vi "Calculator-test_harness.vi"(11 "test case ID":string) -> (3 "result":bool)   [LabVIEW 2018]
doc: "The harness VI is executed for every test case. InstaCoverage passes the test case ID before the execution of the test case in the <b>test case ID</b> input and reads the <b>result</b> output after the execution. If the result is TRUE and no error happens during the execution, then the test case is evaluated as PASSED. If the result is false and no error happens during the execution, then the test case is evaluated as FAILED. Otherwise the test case is evaluated as ERROR.\n\nThe result of the test suite will be PASSED (FAILED) if all (at least one) test cases are PASSED (FAILED). If at least one test case in the test suite has the ERROR result, then the test suite will have ERROR result.\n\n<b>Note: </b>Don't change the connector pane of this VI.\n\nSee the Help Document for more information. (<b>Help</b> > <b>IncQuery Labs</b> > <b>InstaCoverage</b> > <b>InstaCoverage Help...</b>)"
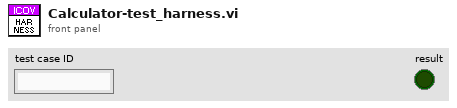
[diagram p1: front panel]
types:
  T1 = typedef "Control 1.ctl" = enum16{"Add", "Subtract", "Multiply", "Divide"}
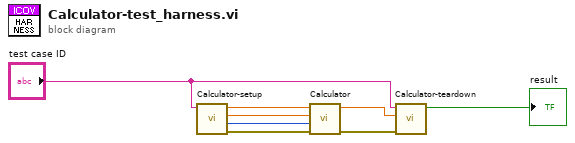
[diagram p0: block diagram]
diagram:
  n1 = call "Calculator-setup.vi"("test case ID"="test case ID") -> ("error out"=w1:errorcluster, "Operation"=w4:T1, "b"=w5:dbl, "a"=w6:dbl)  [unwired: 7 in]
  n2 = call "Calculator.vi"("error in (no error)"=w1, "Operation"=w4, "b"=w5, "a"=w6) -> ("error out"=w3:errorcluster, "result"=w2:dbl)  [unwired: 6 in]
  n3 = call "Calculator-teardown.vi"("error out"=w3, "result"=w2, "test case ID"="test case ID") -> ("result"=→"result":bool)  [unwired: 8 in]
